vi "状态告警区_选择.vi"(10 "Slave ID":u8=1, 11 "data":u16[](array[numeric]) format="%04xH") -> (2 "状态告警区 2":T1, 3 "状态告警区":T2)   [LabVIEW 2016, in "斯坦道总磷总氮.lvlib"]
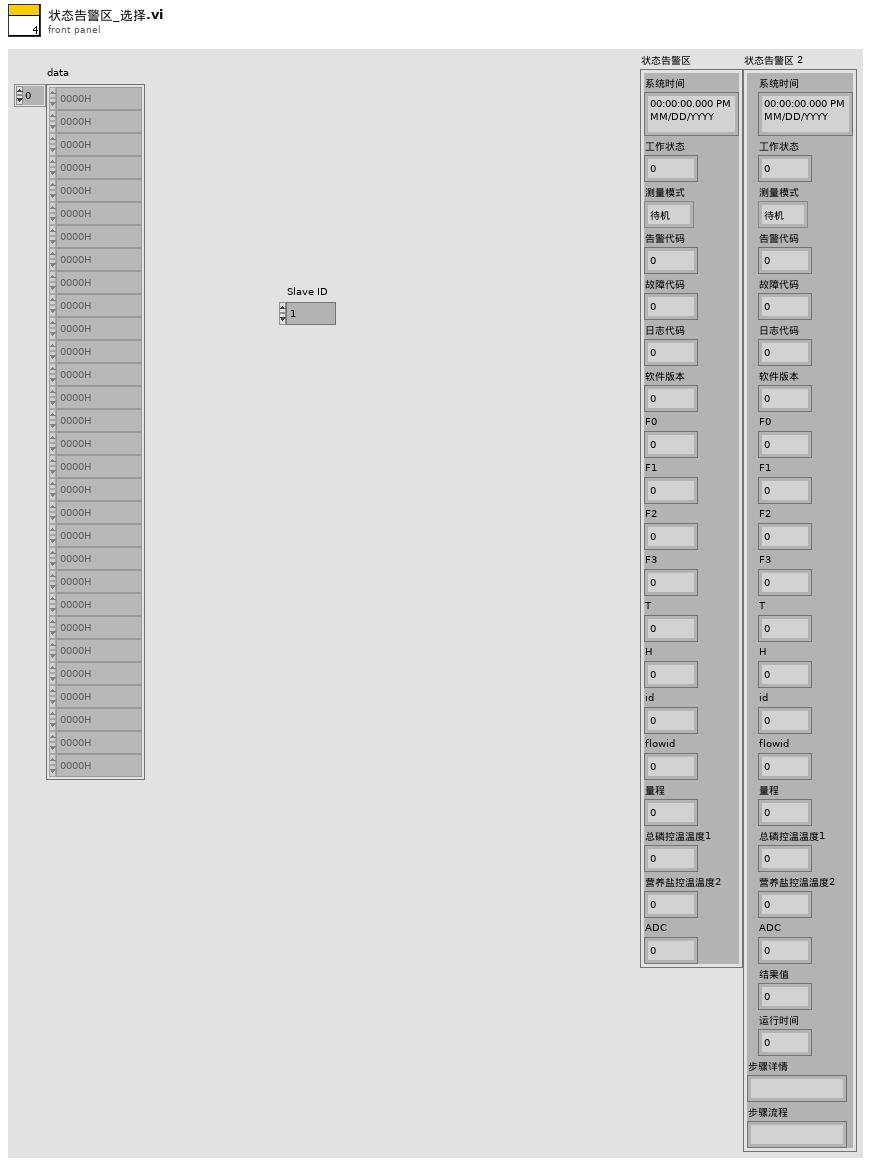
[diagram p1: front panel]
types:
  T1 = cluster{"系统时间":timestamp, "工作状态":u16, "测量模式":enum16{"待机", "连续模式", "周期模式", "定点模式", "受控模式", "手动模式"}, "告警代码":u16, "故障代码":u16, "日志代码":u16, "软件版本":u16, "F0":sgl, "F1":sgl, "F2":sgl, "F3":sgl, "T":sgl, "H":sgl, "id":u16, "flowid":u16, "量程":u16, "总磷控温温度1":sgl, "营养盐控温温度2":sgl, "ADC":sgl, "结果值":sgl, "运行时间":u16, "步骤详情":string, "步骤流程":string}
  T2 = cluster{"系统时间":timestamp, "工作状态":u16, "测量模式":enum16{"待机", "连续模式", "周期模式", "定点模式", "受控模式", "手动模式"}, "告警代码":u16, "故障代码":u16, "日志代码":u16, "软件版本":u16, "F0":sgl, "F1":sgl, "F2":sgl, "F3":sgl, "T":sgl, "H":sgl, "id":u16, "flowid":u16, "量程":u16, "总磷控温温度1":sgl, "营养盐控温温度2":sgl, "ADC":sgl}
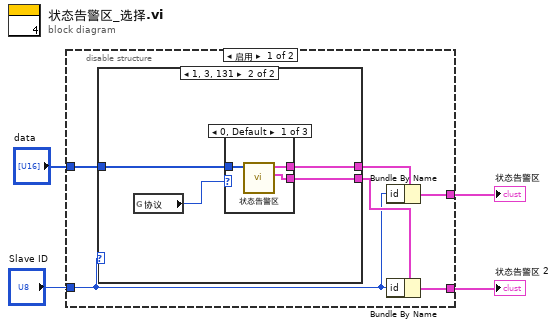
[diagram p0: block diagram]
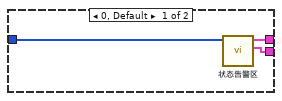
[diagram p2: hidden frame]
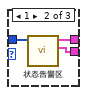
[diagram p3: hidden frame]
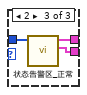
[diagram p4: hidden frame]
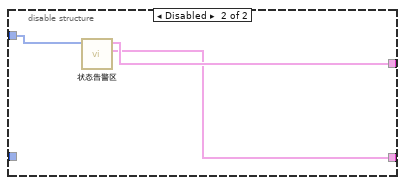
[diagram p5: hidden frame]
diagram:
  n1 = disable-structure shown="启用" {
    disable-tunnel: "data" -> [w10 w29]
    disable-tunnel: [w8 w28] -> w3
    disable-tunnel: "Slave ID" -> [w6 _]
    disable-tunnel: [w5 w27] -> w1
    frame Enabled {
      n2 = case shown="1, 3, 131" w6 {
        tunnel: w10 -> [w13 w17]
        tunnel: [w12 w16] -> w9
        tunnel: [w11 w15] -> w7
        frame 0, Default {
          n3 = call "状态告警区.vi"("数组"=w13) -> ("状态告警区 2"=w11:T1, "状态告警区"=w12:T2)  [unwired: 9 in]
        }
        frame 1, 3, 131 {
          n4 = global read "总磷总氮断电保存全局变量.vi" "协议"() -> (w14:u16)
          n5 = case shown="0, Default" w14 {
            tunnel: w17 -> [w20 w23 w26]
            tunnel: [w19 w22 w25] -> w16
            tunnel: [w18 w21 w24] -> w15
            frame 0, Default {
              n6 = call "状态告警区.vi"("数组"=w20) -> ("状态告警区 2"=w18:T1, "状态告警区"=w19:T2)  [unwired: 9 in]
            }
            frame 1 {
              n7 = call "状态告警区.vi"("数组"=w23) -> ("状态告警区 2"=w21:T1, "状态告警区"=w22:T2)  [unwired: 9 in]
            }
            frame 2 {
              n8 = call "状态告警区_正常.vi"("数组"=w26) -> ("状态告警区 2"=w24:T1, "状态告警区"=w25:T2)  [unwired: 9 in]
            }
          }
        }
      }
      n9 = Bundle By Name(cluster=w9, "id"=w6) -> (w8:T2)
      n10 = Bundle By Name(cluster=w7, "id"=w6) -> (w5:T1)
    }
    frame Disabled {
      n11 = call "状态告警区.vi"("数组"=w29) -> ("状态告警区 2"=w27:T1, "状态告警区"=w28:T2)  [unwired: 9 in]
    }
  }
  "状态告警区" <- w3
  "状态告警区 2" <- w1
